vi "sup_vi_get_marks.vi"() -> (0 "Array":string[][](array[string]))   [LabVIEW 2014]
panel:
  out "cgpa":dbl
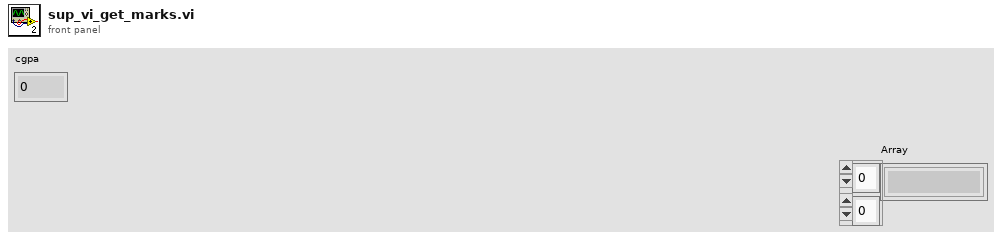
[diagram p1: front panel]
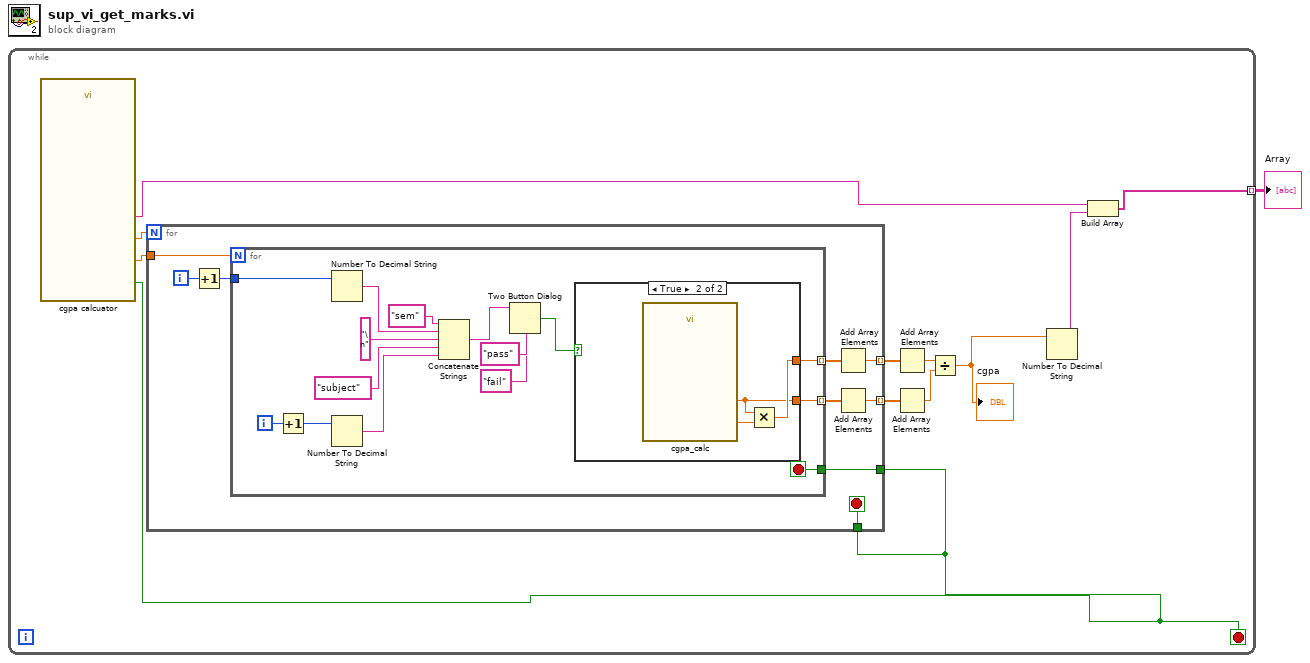
[diagram p0: block diagram]
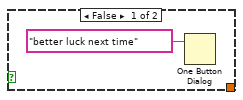
[diagram p2: hidden frame]
diagram:
  n1 = while {
    tunnel: [w3] -> w1 mode=indexing
    stop <- w2 stop-if-true
    n2 = call "cgpa calcuator"() -> ("end of students"=w2:bool, "number of subjects"=w12:dbl, "number of sems"=w11:dbl, "name of student"=w5:string)  [unwired: 14 in, 2 out]
    n3 = for {
      N: w11 -> [_]
      tunnel: w12 -> [w21]
      tunnel: [w17] -> w10 mode=indexing
      tunnel: [w15] -> w9 mode=indexing
      tunnel: w2 -> [w14]
      tunnel: w2 -> [w13]
      i -> [w20]
      stop <- w14 stop-if-true
      n4 = Increment(x=w20) -> (x+1=w19:i32)
      n5 = for {
        N: w21 -> [_]
        tunnel: w19 -> [w36]
        tunnel: [w24] -> w18 mode=indexing
        tunnel: [w23] -> w16 mode=indexing
        tunnel: w13 -> [w22]
        i -> [w35]
        stop <- w22 stop-if-true
        n6 = Increment(x=w35) -> (x+1=w34:i32)
        n7 = Number To Decimal String(number=w36) -> (decimal integer string=w32:string)  [unwired: 1 in]
        n8 = Number To Decimal String(number=w34) -> (decimal integer string=w29:string)  [unwired: 1 in]
        n9 = Concatenate Strings("sem", w32, "\n", "subject", w29) -> (w28:string)
        n10 = Two Button Dialog(message=w28, 1:"fail" ("F button name (\"Cancel\")"), 2:"pass" ("T button name (\"OK\")")) -> (T button?=w25:bool)
        n11 = case shown="True" w25 {
          tunnel: [_ w39] -> w24
          tunnel: [_ w38] -> w23
          frame False {
            n12 = One Button Dialog(message="better luck next time") -> ()  [unwired: 1 in, 1 out]
          }
          frame True {
            n13 = call "cgpa_calc"() -> ("marks"=w40:dbl, "grade points"=w38:dbl)  [unwired: 16 in, 2 out]
            n14 = Multiply(x=w38, y=w40) -> (x*y=w39:dbl)
          }
        }
      }
      n15 = Add Array Elements(numeric array=w18) -> (sum=w17:dbl)
      n16 = Add Array Elements(numeric array=w16) -> (sum=w15:dbl)
    }
    n17 = Add Array Elements(numeric array=w10) -> (sum=w8:dbl)
    n18 = Add Array Elements(numeric array=w9) -> (sum=w7:dbl)
    n19 = Divide(x=w8, y=w7) -> (x/y=w6:dbl)
    "cgpa" <- w6
    n20 = Number To Decimal String(number=w6) -> (decimal integer string=w4:string)  [unwired: 1 in]
    n21 = Build Array(w5, w4) -> (w3:string[])
  }
  "Array" <- w1
